vi "Read Read.vi"(8 "error in (no error)":errorcluster, 11 "myOtherClass in":refnum<class "myOtherClass.lvclass">) -> (0 "error out":errorcluster, 2 "Read":bool, 3 "myOtherClass out":refnum<class "myOtherClass.lvclass">)   [LabVIEW 2017, in "myOtherClass.lvclass"]
uses:
  myOtherClass.lvclass
  myOtherClass.lvclass/myOtherClass.ctl
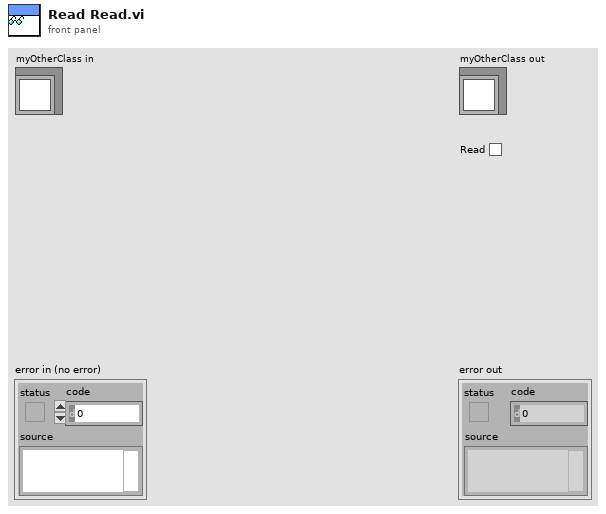
[diagram p1: front panel]
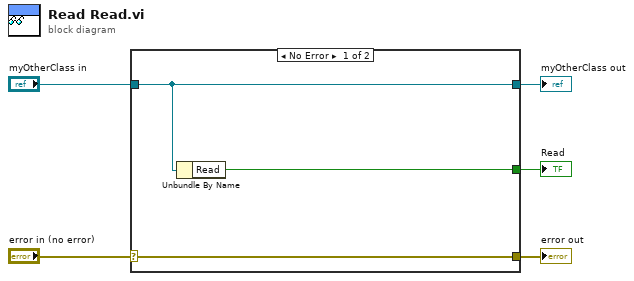
[diagram p0: block diagram]
diagram:
  n1 = case shown="No Error" "error in (no error)" {
    selector: "error in (no error)" -> [w8 w9]
    tunnel: [w8 w9] -> w4
    tunnel: [w7 w10] -> w2
    tunnel: "myOtherClass in" -> [w7 w10]
    tunnel: [w6 _] -> w1
    frame No Error {
      n2 = Unbundle By Name(w7) -> ("Read"=w6:bool)
    }
    frame Error {
    }
  }
  "error out" <- w4
  "myOtherClass out" <- w2
  "Read" <- w1
